vi "TDC Tester.vi"() -> ()   [LabVIEW 2014]
doc: "TDC Tester"
uses:
  FA_TDC.lvlib
  FA_NativeTypes API/source/VI Source/FA_NativeTypes.lvlib
  FA_LocalStore API/source/VI Source/FA_LocalStore.lvlib
  FA_LocalStore API/source/VI Source/FA_LSSpecialTypes.ctl
  FA_TDC.ctl
panel:
  out "TDC 2":T1
  out "Error Out":errorcluster
  in  "Error In":errorcluster
  in  "TDC":T1={"API Key"="myAPIkey", "Private Key"="myPrivatekey", "Base URL"="myBaseURL", "Channels"=[{"Channel URL"="a", "Start Time"=timestamp(3426008619 s since 1904-01-01), "End Time"=timestamp(3426008621.912 s since 1904-01-01), "Number of Values"=1}, {"Channel URL"="b", "Start Time"=timestamp(3426095027.95 s since 1904-01-01), "End Time"=timestamp(3426095030.931 s since 1904-01-01), "Number of Values"=2}]}
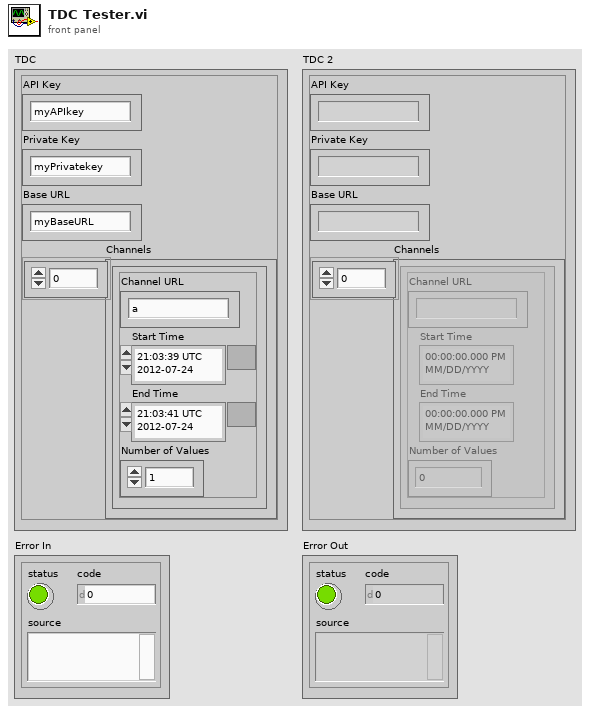
[diagram p1: front panel]
types:
  T1 = typedef "FA_TDC.lvlib/FA_TDC.ctl" = cluster{"API Key":string, "Private Key":string, "Base URL":string, "Channels":cluster{"Channel URL":string, "Start Time":timestamp, "End Time":timestamp, "Number of Values":i32}[]}
  T2 = typedef "FA_LocalStore.lvlib/FA_LSSpecialTypes.ctl" = string
  T3 = typedef "FA_NativeTypes.lvlib/FA_Config.ctl" = cluster{"Id":string, "Name":T2, "Parameter":cluster{"Name":string, "Value":string}[], "Account":string, "CreateDate":string, "LastModified":string}
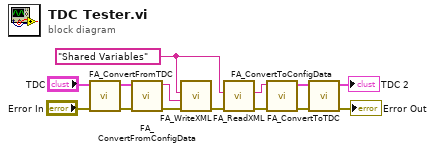
[diagram p0: block diagram]
diagram:
  w4 = T2 "Shared Variables" ("Special Type")
  n1 = call "FA_ConvertFromTDC.vi"("Error In"="Error In", "TDC"="TDC") -> ("Error Out"=w11:errorcluster, "Config"=w12:T3)  [unwired: 8 in]
  n2 = call "FA_ConvertFromConfigData.vi"("Error In"=w11, "Config"=w12) -> ("Error Out"=w7:errorcluster, "XML String"=w6:string)  [unwired: 8 in]
  n3 = call "FA_WriteXML.vi"("Error In"=w7, "XML String"=w6, "Special Type"=w4) -> ("Error Out"=w5:errorcluster)  [unwired: 6 in]
  n4 = call "FA_ReadXML.vi"("Error In"=w5, "Special Type"=w4) -> ("Error Out"=w2:errorcluster, "XML String"=w3:string)  [unwired: 6 in]
  n5 = call "FA_ConvertToConfigData.vi"("Error In"=w2, "XML String"=w3) -> ("Error Out"=w9:errorcluster, "ConfigData"=w10:T3)  [unwired: 8 in]
  n6 = call "FA_ConvertToTDC.vi"("Error In"=w9, "Config"=w10) -> ("Error Out"=→"Error Out":errorcluster, "TDC"=→"TDC 2":T1)  [unwired: 8 in]
